vi "chaos-ui-test.vi"() -> ()   [LabVIEW 2012, in "chaosui-crest.lvlib"]
uses:
  chaosui-crest.lvlib
  ChaosDevState.ctl
panel:
  out "dev_state":T1
  out "dev_state_out 2":T1
  out "dev_error":bool
  out "loop":i32
  in  "milliseconds to wait":u32=500
  in  "stop":bool
  out "timestamp":u64
  out "nok":i32
  out "output out":string
  in  "timeout (10000)":i32=10000
  in  "cuname":string
  in  "chaoswanurl":string="chaost-webui1.chaos.lnf.infn.it:8081"
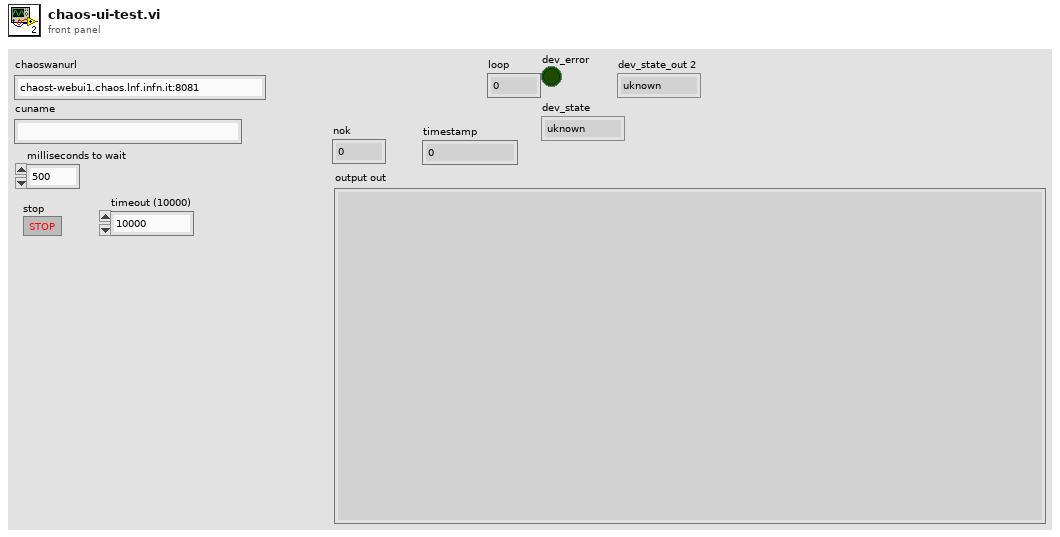
[diagram p1: front panel]
types:
  T1 = typedef "ChaosDevState.ctl" = enum16{"uknown", "stop", "init", "deinit", "start"}
  T2 = typedef "LabVIEWHTTPClient.lvlib/ClientHandle.ctl" = refnum<k1>
  T3 = cluster{"client handle out":T2, "chaoswanurl":string}
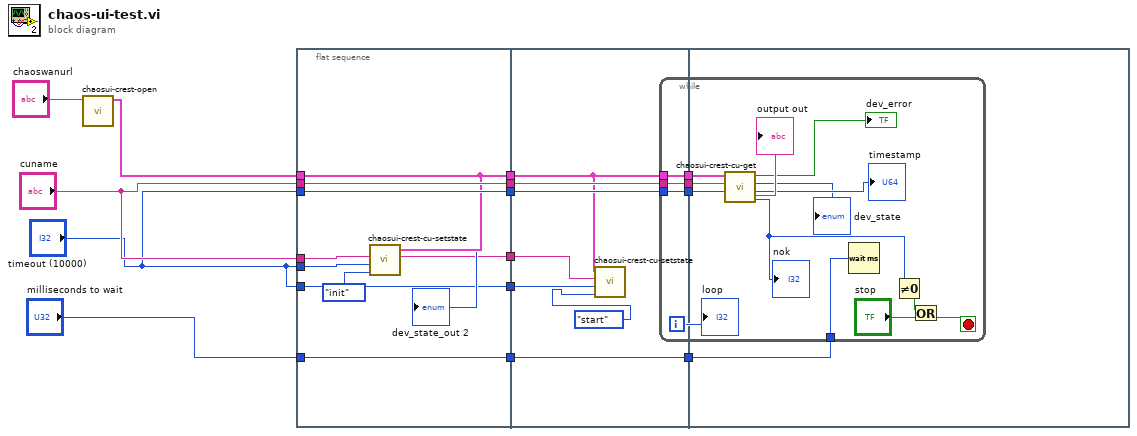
[diagram p0: block diagram]
diagram:
  n1 = call "chaosui-crest-open.vi"("chaoswanurl"="chaoswanurl") -> ("handle"=w13:T3)  [unwired: 10 in]
  n2 = flat-sequence {
    tunnel: "timeout (10000)" -> [w22]
    tunnel: "cuname" -> [w23]
    tunnel: w13 -> [w20]
    tunnel: "milliseconds to wait" -> [w24]
    tunnel: [w24] -> w11
    tunnel: [w20] -> w9
    tunnel: [w23] -> w7
    tunnel: [w22] -> w5
    tunnel: "cuname" -> [w18]
    tunnel: "timeout (10000)" -> [w21]
    tunnel: [w18] -> w3
    tunnel: "timeout (10000)" -> [w17]
    tunnel: [w17] -> w1
    tunnel: w11 -> [w31]
    tunnel: [w31] -> w10
    tunnel: w9 -> [w27]
    tunnel: [w27] -> w8
    tunnel: w7 -> [w30]
    tunnel: [w30] -> w6
    tunnel: w5 -> [w29]
    tunnel: [w29] -> w4
    tunnel: w3 -> [w28]
    tunnel: w1 -> [w26]
    tunnel: w10 -> [w35]
    tunnel: w8 -> [w34]
    tunnel: w6 -> [w33]
    tunnel: w4 -> [w32]
    frame #0 {
      n3 = call "chaosui-crest-cu-setstate.vi"("dev_state"=ChaosDevState."init", "timeout (10000)"=w21, "cuname"=w18, "handleConnection"=w20) -> ("dev_state_out"=→"dev_state_out 2":T1)  [unwired: 4 out]
    }
    frame #1 {
      n4 = call "chaosui-crest-cu-setstate.vi"("dev_state"=ChaosDevState."start", "timeout (10000)"=w26, "cuname"=w28, "handleConnection"=w27) -> ()  [unwired: 5 out]
    }
    frame #2 {
      n5 = while {
        tunnel: w34 -> [w48]
        tunnel: w33 -> [w47]
        tunnel: w32 -> [w46]
        tunnel: w35 -> [w43]
        i -> [w42]
        stop <- w39 stop-if-true
        n6 = call "chaosui-crest-cu-get.vi"("timeout (10000)"=w46, "cuname"=w47, "handleConnection"=w48) -> ("nok"=w38:i32, "timestamp"=→"timestamp":u64, "dev_state"=→"dev_state":T1, "dev_error"=→"dev_error":bool, "output out"=→"output out":string)  [unwired: 2 in]
        "nok" <- w38
        n7 = Wait (ms)(milliseconds to wait=w43) -> ()  [unwired: 1 out]
        n8 = Not Equal To 0?(x=w38) -> (x != 0?=w37:bool)
        n9 = Or(x=w37, y="stop") -> (x .or. y?=w39:bool)
        "loop" <- w42
      }
    }
  }
